vi "READINGbinary.vi"() -> ()   [LabVIEW 2023]
panel:
  out "data":dbl
  in  "file path (use dialog)":path
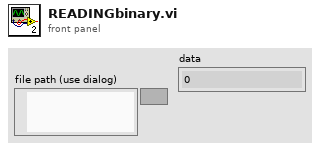
[diagram p1: front panel]
types:
  T1 = enum16{"open", "replace", "create", "open or create", "replace or create", "replace or create with confirmation"}
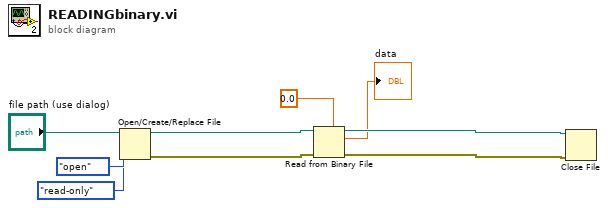
[diagram p0: block diagram]
diagram:
  n1 = Open/Create/Replace File(file path (use dialog)="file path (use dialog)", operation (0:open)=T1."open", access (0:read/write)=enum16{"read/write", "read-only", "write-only"}."read-only") -> (refnum out=w9:refnum<file>, error out=w8:errorcluster)  [unwired: 3 in, 1 out]
  n2 = Read from Binary File(5:0.0, 8:w8, 11:w9) -> (0:w6:errorcluster, 2:→"data":dbl, 3:w7:refnum<file>)  [unwired: 3 in, 1 out]
  n3 = Close File(refnum=w7, error in=w6) -> ()  [unwired: 2 out]
